vi "Get Put Updater.vi"(7 "Select":enum16{"Get", "Put"}(ring), 8 "에러 입력(에러 없음)":errorcluster) -> (0 "에러 출력":errorcluster)   [LabVIEW 2020]
uses:
  Controls/Cmd_File path.ctl
  <vilib>/FTP/NI_FTP.lvlib
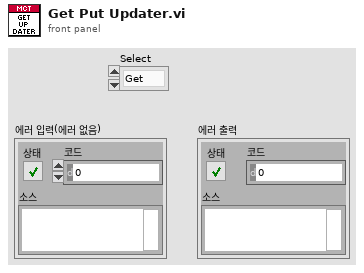
[diagram p1: front panel]
types:
  T1 = typedef "Cmd_File path.ctl" = enum16{"에러로그", "데이터파일경로", "성적서원본", "지난성적서", "Data Files", "경로생성", "Updater", "Template", "설정파일경로", "FTP Upload", "Update 경로", "어플리케이션"}
  T2 = enum32{"invalid app kind", "Development System", "Run Time System", "Student Edition", "Embedded LabVIEW", "Evaluation", "Custom"}
  T3 = typedef "NI_FTP.lvlib/FTP Session.ctl" = refnum<k5>
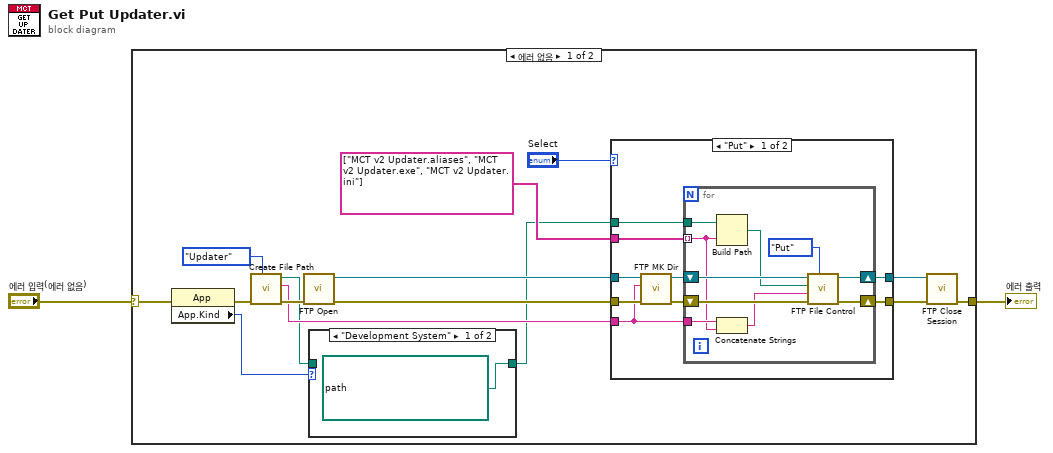
[diagram p0: block diagram]
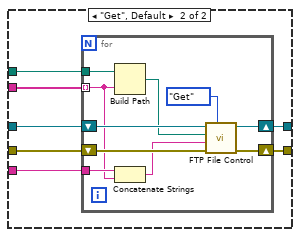
[diagram p3: hidden frame]
diagram:
  n1 = case shown="에러 없음" "에러 입력(에러 없음)" {
    selector: "에러 입력(에러 없음)" -> [w7 w56]
    tunnel: [w15 w56] -> w2
    frame No Error {
      n2 = property class="App"(error in=w7) -> (error out=w6:errorcluster, "App.Kind"=w5:T2)  [unwired: 1 in, 1 out]
      n3 = call "Create File Path.vi"("항목"=Cmd_File_path."Updater", "에러 입력"=w6) -> ("error out"=w9:errorcluster, "문자열 out"=w8:string, "파일경로"=w4:path)  [unwired: 6 in, 1 out]
      n4 = call "FTP Open.vi"("에러 입력(에러 없음)"=w9) -> ("에러 출력"=w12:errorcluster, "TCP 네트워크 연결 출력"=w13:T3)  [unwired: 9 in]
      n5 = case shown="\"Development System\"" w5 {
        tunnel: w4 -> [_ w19]
        tunnel: [path "D:/Jey/OneDrive/문서/업무_개발/Calibration Tool Project/builds/MCT v2/MCT v2 Updater" w19] -> w3
        frame "Development System" {
        }
        frame Default {
        }
      }
      n6 = case shown="\"Put\"" "Select" {
        tunnel: w8 -> [w21 w39]
        tunnel: string[] ["MCT v2 Updater.aliases", "MCT v2 Updater.exe", "MCT v2 Updater.ini"] -> [w28 w45]
        tunnel: w3 -> [w20 w44]
        tunnel: [w27 w43] -> w16
        tunnel: [w26 w42] -> w14
        tunnel: w13 -> [w24 w41]
        tunnel: w12 -> [w25 w40]
        frame "Put" {
          n7 = call "FTP MK Dir.vi"("에러 입력(에러 없음)"=w25, "디렉토리명"=w21, "ftp session"=w24) -> ("에러 출력"=w22:errorcluster, "ftp session out"=w23:T3)  [unwired: 7 in]
          n8 = for {
            shift-right: [w36] -> w26
            shift-left: w22 -> [w38]
            shift-right: [w35] -> w27
            shift-left: w23 -> [w37]
            tunnel: w20 -> [w34]
            tunnel: w28 -> [w32] mode=indexing
            tunnel: w21 -> [w33]
            n9 = Build Path(base path=w34, name or relative path=w32) -> (appended path=w30:path)
            n10 = Concatenate Strings(w33, w32) -> (w29:string)
            n11 = call "FTP File Control.vi"("Comm"=enum16{"Get", "Put"}."Put", "에러 입력"=w38, "원격경로"=w29, "로컬경로"=w30, "TCP 네트워크 연결 입력"=w37) -> ("에러 출력"=w36:errorcluster, "TCP 네트워크 연결 출력"=w35:T3)  [unwired: 2 in, 3 out]
          }
        }
        frame "Get", Default {
          n12 = for {
            shift-right: [w53] -> w42
            shift-left: w40 -> [w55]
            shift-right: [w52] -> w43
            shift-left: w41 -> [w54]
            tunnel: w44 -> [w51]
            tunnel: w45 -> [w49] mode=indexing
            tunnel: w39 -> [w50]
            n13 = Build Path(base path=w51, name or relative path=w49) -> (appended path=w47:path)
            n14 = Concatenate Strings(w50, w49) -> (w46:string)
            n15 = call "FTP File Control.vi"("Comm"=enum16{"Get", "Put"}."Get", "에러 입력"=w55, "원격경로"=w46, "로컬경로"=w47, "TCP 네트워크 연결 입력"=w54) -> ("에러 출력"=w53:errorcluster, "TCP 네트워크 연결 출력"=w52:T3)  [unwired: 2 in, 3 out]
          }
        }
      }
      n16 = call <vilib>:"FTP Close Session.vi"("error in (no error)"=w14, "ftp session"=w16) -> ("error out"=w15:errorcluster)  [unwired: 6 in, 3 out]
    }
    frame Error {
    }
  }
  "에러 출력" <- w2
